vi "Start Module.vi"(8 "error in (no error)":errorcluster, 10 "Sequence Context In":refnum<k7>) -> (0 "error out":errorcluster, 1 "Wait for Event Sync?":bool, 2 "TestStand Manager_DQMH Broadcast Events":T1)   [LabVIEW 2015, in "TestStand Manager_DQMH.lvlib"]
doc: "Launches the Module Main.vi.\n_____\nBased on Delacor QMH Project Template 2.0.0.62.\n____\nDelacor QMH Thermal Chamber Examples 4.0.0.21\nCopyright (c) 2018, Delacor"
uses:
  TestStand Manager_DQMH.lvlib
  Broadcast Events--cluster.ctl
  Did Init Argument--cluster.ctl
  Status Updated Argument--cluster.ctl
  Error Reported Argument--cluster.ctl
  Stop Argument--cluster.ctl
  Get Module Execution Status Argument--cluster.ctl
  <vilib>/Delacor/Delacor QMH/Libraries/Module Admin_class/Delacor_lib_QMH_Module Admin.lvclass
  <vilib>/Delacor/Delacor QMH/Libraries/Module Admin_class/Delacor_lib_QMH_Module Admin.lvclass/Delacor_lib_QMH_Module Admin.ctl
  <vilib>/Delacor/Delacor QMH/Libraries/Module Admin_class/Delacor_lib_QMH_Set External Launch.vi
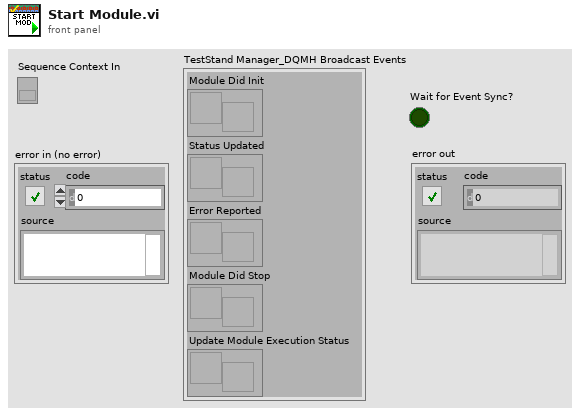
[diagram p1: front panel]
types:
  T1 = typedef "TestStand Manager_DQMH.lvlib/Broadcast Events--cluster.ctl" = cluster{"Module Did Init":refnum<user-event>, "Status Updated":refnum<user-event>, "Error Reported":refnum<user-event>, "Module Did Stop":refnum<user-event>, "Update Module Execution Status":refnum<user-event>}
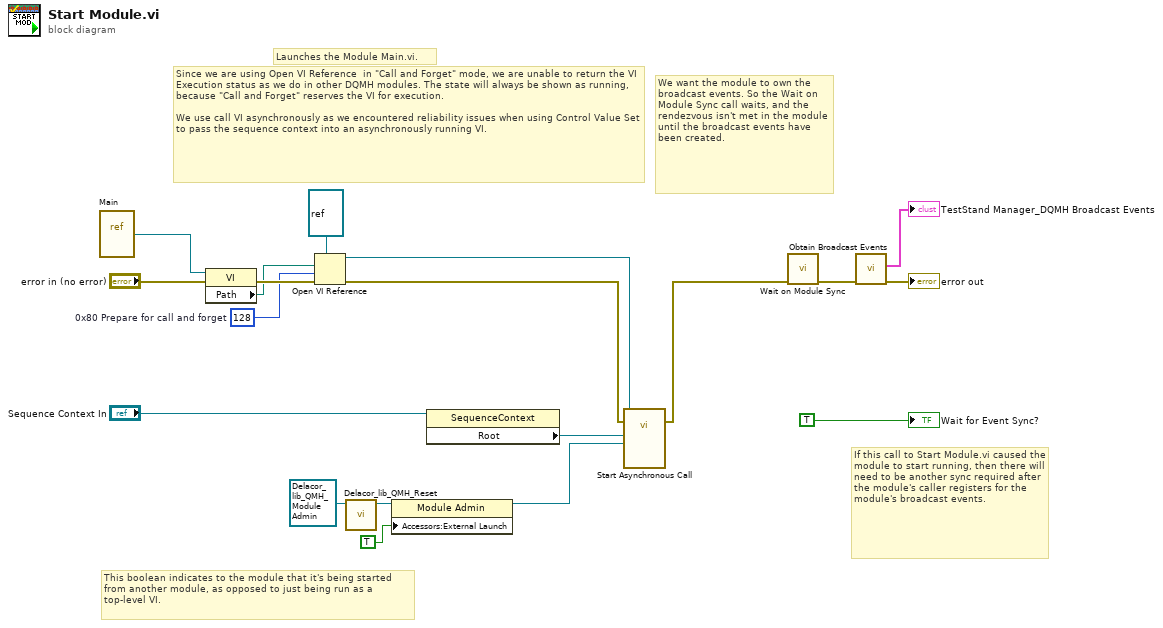
[diagram p0: block diagram]
diagram:
  w4 = 128  # 0x80 Prepare for call and forget
  # "Since we are using Open VI Reference  in \"Call and Forget\" mode, we are unable to return the VI Execution status as we do in other DQMH modules. The state will always be shown as running, because \"Call and Forget\" reserves the VI for execution.\n\nWe use call VI asynchronously as we encountered reliability issues when using Control Value Set to pass the sequence context into an asynchronously running VI."
  # "We want the module to own the broadcast events. So the Wait on Module Sync call waits, and the rendezvous isn't met in the module until the broadcast events have been created."
  # "This boolean indicates to the module that it's being started from another module, as opposed to just being run as a top-level VI."
  # "If this call to Start Module.vi caused the module to start running, then there will need to be another sync required after the module's caller registers for the module's broadcast events."
  # "Launches the Module Main.vi."
  n1 = vi-ref "Main.vi"() -> (w19:refnum<vi>)
  n2 = property class="VI"(reference=w19, error in="error in (no error)") -> (error out=w10:errorcluster, "Path"=w7:path)  [unwired: 1 out]
  n3 = Open VI Reference(type specifier VI Refnum (for type only)=refnum<vi> refnum, vi path=w7, options=w4, error in (no error)=w10) -> (vi reference=w6:refnum<vi>, error out=w8:errorcluster)  [unwired: 2 in]
  n4 = call-dynamic "Delacor_lib_QMH_Reset.vi"("Mod Admin in"=refnum<class "Delacor_lib_QMH_Module Admin.lvclass"> refnum) -> ("Mod Admin out"=w13:refnum<class "Delacor_lib_QMH_Module Admin.lvclass">)  [unwired: 9 in, 1 out]
  n5 = property class="Module Admin"(reference=w13, "Accessors:External Launch"=TRUE) -> (reference out=w3:refnum<class "Delacor_lib_QMH_Module Admin.lvclass">)  [unwired: 1 in, 1 out]
  n6 = property class="SequenceContext"(reference="Sequence Context In") -> ("Root"=w1:refnum<k7>)  [unwired: 1 in, 2 out]
  n7 = call-by-ref "Start Asynchronous Call"(reference=w6, error in=w8, "Module Admin"=w3, "Sequence Context In"=w1) -> (error out=w9:errorcluster)  [unwired: 10 in, 1 out]
  n8 = call "Wait on Module Sync.vi"("error in (no error)"=w9) -> ("error out"=w17:errorcluster)  [unwired: 10 in]
  n9 = call "Obtain Broadcast Events.vi"("error in (no error)"=w17) -> ("error out"=→"error out":errorcluster, "TestStand Manager_DQMH Broadcast Events"=→"TestStand Manager_DQMH Broadcast Events":T1)  [unwired: 9 in]
  "Wait for Event Sync?" <- TRUE
